vi "IDW Receive - Multi Byte.vi"() -> ()   [LabVIEW 2009]
doc: "An example program for the I2C Digital Waveform library. This VI constructs a simple master-receiver waveform for a multi-byte read operation on an I2C bus."
uses:
  user.lib/I2C Digital Waveform/_Typedefs/Timing - ns.ctl
  user.lib/I2C Digital Waveform/_Typedefs/Bus mode.ctl
  user.lib/I2C Digital Waveform/_Typedefs/Bit type.ctl
  user.lib/I2C Digital Waveform/_Polymorphics/Init - Preallocate.vi
  user.lib/I2C Digital Waveform/_Typedefs/Bus operation.ctl
  user.lib/I2C Digital Waveform/_Typedefs/Start action.ctl
  user.lib/I2C Digital Waveform/_Typedefs/ACK action.ctl
  user.lib/I2C Digital Waveform/IDW.lvlib
panel:
  out "Compare bits":cluster{"Locations":u64[], "Types":T1[]}
  in  "Sample quantum (min 1)":i32=2 caption="Sample quantum \nmin 1)" min=1
  in  "Samples to allocate":i32=100000 format="%.0p"
  out "Coerced timing (ns)":T2 {"fSCL" format="%#_6p"}
  out "I2C digital waveform":digitalwaveform(graph)
  in  "Sample rate":dbl=100000000.0 format="%#_6p"
  in  "Mode":T3="Standard-mode"
  in  "I2C timing (ns)":T2={"tSU;STA"=4700, "tHD;STA"=4000, "tSU;DAT"=250, "tHD;DAT"=5000, "tSU;STO"=4000, "tBUF"=4700, "tHIGH"=4000, "fSCL"=100000.0} {"fSCL" format="%#_6p"}
  in  "Expected data":u8[](array[numeric])=[1, 35, 69, 103] format="%02x"
  in  "Slave address":u8=170 format="%02x"
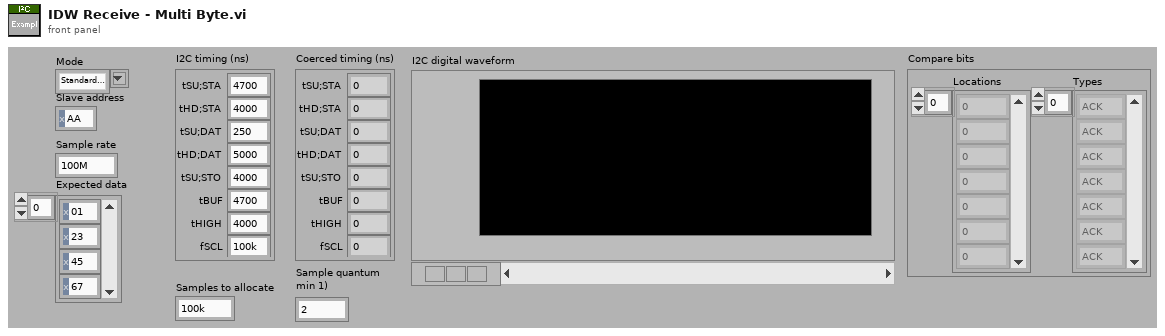
[diagram p1: front panel]
types:
  T1 = typedef "IDW.lvlib/Bit type.ctl" = enum16{"ACK", "Data"}
  T2 = typedef "IDW.lvlib/Timing - ns.ctl" = cluster{"tSU;STA":i32, "tHD;STA":i32, "tSU;DAT":i32, "tHD;DAT":i32, "tSU;STO":i32, "tBUF":i32, "tHIGH":i32, "fSCL":dbl}
  T3 = typedef "IDW.lvlib/Bus mode.ctl" = string
  T4 = cluster{"tSU;STA":bool, "tHD;STA":bool, "tSU;DAT":bool, "tHD;DAT":bool, "tSU;STO":bool, "tBUF":bool, "tHIGH":bool, "fSCL":bool}
  T5 = typedef "IDW.lvlib/Start action.ctl" = enum16{"S", "Sr"}
  T6 = typedef "IDW.lvlib/ACK action.ctl" = enum16{"Listen ACK", "Listen NACK", "Send ACK", "Send NACK"}
  T7 = typedef "IDW.lvlib/Bus operation.ctl" = enum16{"Tx", "Rx"}
  T8 = typedef "IDW.lvlib/Waveform info.ctl" = cluster{"Last sample":u8[], "Sample offset":u64, "Compare offset":u64, "Timing (ticks)":T9, "Preallocated":bool, "Def trans action":T10, "Data Q":refnum<queue>, "Comp types Q":refnum<queue>, "Comp locs Q":refnum<queue>}
  T9 = typedef "IDW.lvlib/Timing - ticks.ctl" = cluster{"tSU;STA":i32, "tHD;STA":i32, "tSU;DAT":i32, "tHD;DAT":i32, "tSU;STO":i32, "tBUF":i32, "tHIGH":i32, "Trans length":i32, "0-30 Rise":i32, "0-70 Rise":i32, "100-30 Fall":i32}
  T10 = typedef "IDW.lvlib/Default transition action.ctl" = enum16{"Hold low (0)", "Release (Z)", "Set up next value", "Hold previous value", "Preserve tHD;DAT and tSU;DAT"}
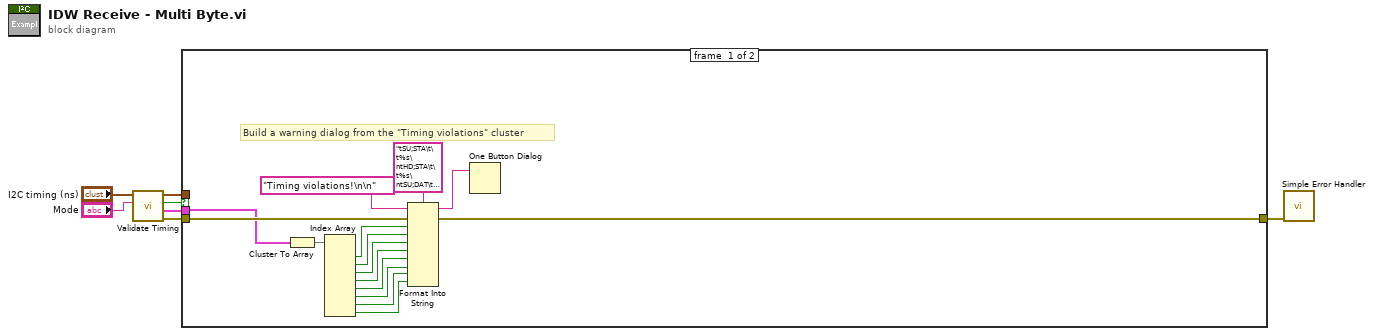
[diagram p0: block diagram]
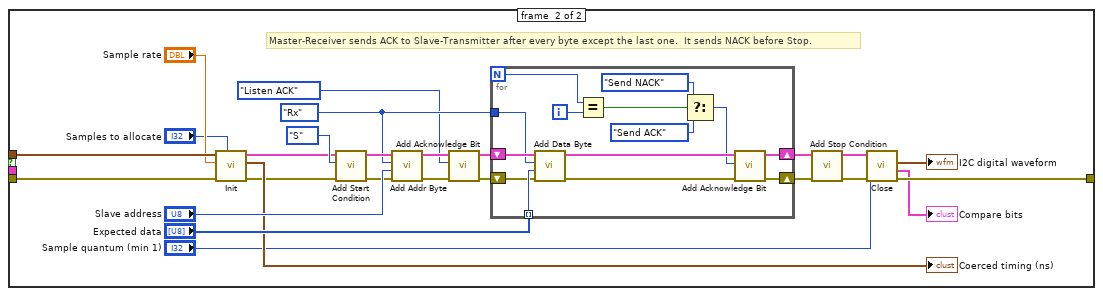
[diagram p2: hidden frame]
diagram:
  n1 = call "Validate Timing.vi"("Mode"="Mode", "I2C timing (ns)"="I2C timing (ns)") -> ("error out"=w2:errorcluster, "Timing violations"=w3:T4, "Timing passed?"=w4:bool, "I2C timing (ns) out"=w7:T2)  [unwired: 1 in, 5 out]
  n2 = case shown="True" w4 {
    tunnel: w7 -> [_ w31]
    tunnel: w3 -> [w8 _]
    tunnel: w2 -> [w10 w26]
    tunnel: [w9 w38] -> w1
    frame #0 {
      # "Build a warning dialog from the \"Timing violations\" cluster"
      n3 = Cluster To Array(cluster=w8) -> (array=w22:bool[])
      n4 = Index Array(array=w22) -> (element #1=w21:bool, element #2=w20:bool, element #3=w19:bool, element #4=w18:bool, element #5=w17:bool, element #6=w16:bool, element #7=w15:bool, element #8=w14:bool)  [unwired: 8 in]
      n5 = Format Into String(format string="tSU;STA\t\t%s\ntHD;STA\t\t%s\ntSU;DAT\t\t%s\ntHD;DAT\t\t%s\ntSU;STO\t\t%s\ntBUF\t\t%s\ntHIGH\t\t%s\nfSCL\t\t%s", initial string="Timing violations!\n\n", error in=w10, w21, w20, w19, w18, w17, w16, w15, w14) -> (resulting string=w11:string, error out=w9:errorcluster)
      n6 = One Button Dialog(message=w11) -> ()  [unwired: 2 out]
    }
    frame #1 {
      w42 = Bus_operation."Rx" ("Bus operation")
      # "Master-Receiver sends ACK to Slave-Transmitter after every byte except the last one.  It sends NACK before Stop."
      n7 = call-poly "Init.vi"("Samples to allocate"="Samples to allocate", "error in (no error)"=w26, "Sample rate"="Sample rate", "I2C timing (ns)"=w31) -> ("error out"=w27:errorcluster, "Coerced I2C timing (ns)"=→"Coerced timing (ns)":T2, "I2C waveform info"=w29:T8)  [unwired: 1 in, 4 out]
      n8 = call "Add Start Condition.vi"("error in (no error)"=w27, "Action"=Start_action."S", "I2C waveform info"=w29) -> ("error out"=w37:errorcluster, "I2C waveform info out"=w48:T8)  [unwired: 1 in, 6 out]
      n9 = call "Add Addr Byte.vi"("error in (no error)"=w37, "Slave address"="Slave address", "Bus operation"=w42, "I2C waveform info"=w48) -> ("error out"=w36:errorcluster, "I2C waveform info out"=w47:T8)  [unwired: 6 out]
      n10 = call "Add Acknowledge Bit.vi"("error in (no error)"=w36, "Action"=ACK_action."Listen ACK", "I2C waveform info"=w47) -> ("error out"=w35:errorcluster, "I2C waveform info out"=w46:T8)  [unwired: 7 out]
      n11 = for {
        N -> [w53]
        tunnel: "Expected data" -> [w59] mode=indexing
        tunnel: w42 -> [w58]
        shift-right: [w60] -> w45
        shift-left: w46 -> [w62]
        shift-right: [w55] -> w34
        shift-left: w35 -> [w57]
        i -> [w54]
        n12 = call "Add Data Byte.vi"("error in (no error)"=w57, "Data"=w59, "Action"=w58, "I2C waveform info"=w62) -> ("error out"=w56:errorcluster, "I2C waveform info out"=w61:T8)  [unwired: 6 out]
        n13 = Equal?(x=w53, y=w54) -> (x = y?=w52:bool)
        n14 = Select(t=ACK_action."Send NACK" ("Action"), s=w52, f=ACK_action."Send ACK" ("Action")) -> (s? t:f=w49:T6)
        n15 = call "Add Acknowledge Bit.vi"("error in (no error)"=w56, "Action"=w49, "I2C waveform info"=w61) -> ("error out"=w55:errorcluster, "I2C waveform info out"=w60:T8)  [unwired: 7 out]
      }
      n16 = call "Add Stop Condition.vi"("error in (no error)"=w34, "I2C waveform info"=w45) -> ("error out"=w33:errorcluster, "I2C waveform info out"=w40:T8)  [unwired: 8 out]
      n17 = call "Close.vi"("error in (no error)"=w33, "Sample quantum (min 1)"="Sample quantum (min 1)", "I2C waveform info"=w40) -> ("error out"=w38:errorcluster, "Compare bits"=→"Compare bits":cluster{"Locations":u64[], "Types":T1[]}, "Dig waveform out"=→"I2C digital waveform":digitalwaveform)  [unwired: 1 in, 5 out]
    }
  }
  n18 = call <vilib>:"Simple Error Handler.vi"("error in (no error)"=w1) -> ()  [unwired: 1 in, 8 out]
